vi "Default Secret Configuration--constant.vi"() -> (3 "Path":path)   [LabVIEW 2025]
doc: "This constant defines the path to the standard configuration XML file."
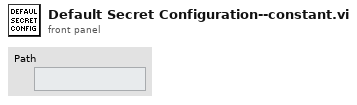
[diagram p1: front panel]
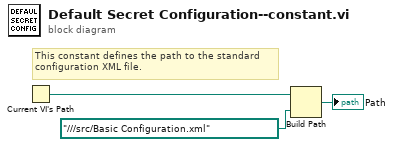
[diagram p0: block diagram]
diagram:
  # "This constant defines the path to the standard\nconfiguration XML file."
  n1 = Current VI's Path() -> (path=w1:path)
  n2 = Build Path(base path=w1, name or relative path=path "../../../src/Basic Configuration.xml") -> (appended path=→"Path":path)
